vi "Device Label to Configuration.vi"(8 "error in (no error)":errorcluster, 10 "Ring Labels":string[](array[string]), 11 "UI in":T1 {"KH"."Channel" items=["A 1"]}) -> (0 "error out":errorcluster, 3 "UI out":T1 {"KH"."Channel" items=["A 1"]})   [LabVIEW 2016, in "Control Experiment UI.lvclass"]
uses:
  Control Experiment UI.lvclass
  Typedefs/UI Channels--Cluster.ctl
  Typedefs/UI Channels.AI--Cluster.ctl
  Typedefs/UI Channels.Device--Cluster.ctl
  Control Experiment SM/Typedefs/KH Mode-enum.ctl
  Typedefs/UI Channels.KH--Cluster.ctl
  <userlib>/LevyLab/Krohn Hite 7008/typedefs/Input Configuration-Enum.ctl
  <userlib>/LevyLab/Krohn Hite 7008/typedefs/Gain-Enum.ctl
  <userlib>/LevyLab/Krohn Hite 7008/typedefs/Shunt-Enum.ctl
  Typedefs/UI Channels.AO--Cluster.ctl
  <userlib>/LevyLab/Krohn Hite 7008/Instrument.KH7008.lvclass
  Control Experiment SM/Control Experiment SM.lvclass
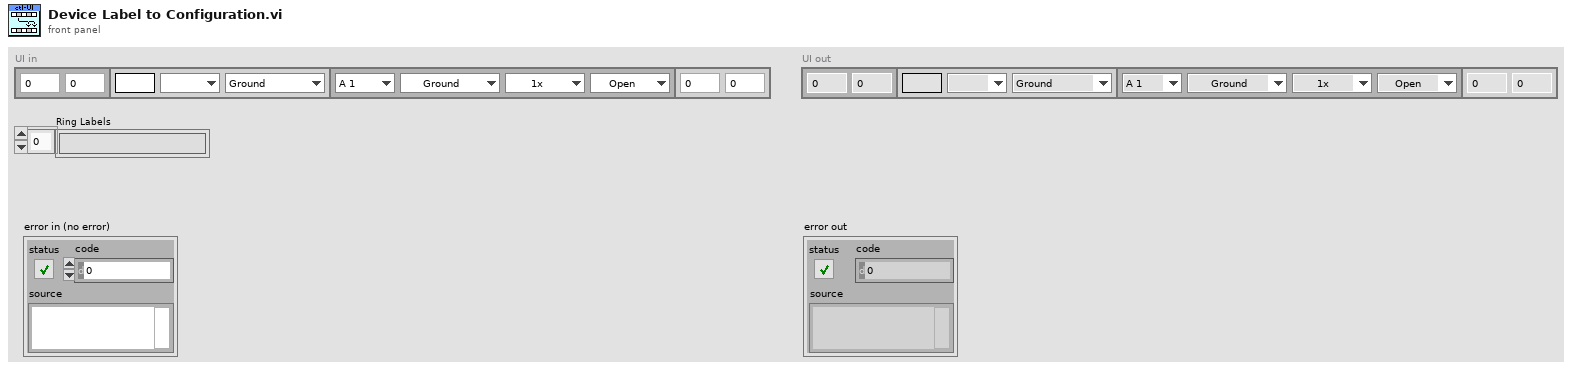
[diagram p1: front panel]
types:
  T1 = typedef "Control Experiment UI.lvclass/UI Channels--Cluster.ctl" = cluster{"AI":T2, "Device":T3, "KH":T5, "AO":T9}
  T2 = typedef "Control Experiment UI.lvclass/UI Channels.AI--Cluster.ctl" = cluster{"Channel":u32, "Gain":dbl}
  T3 = typedef "Control Experiment UI.lvclass/UI Channels.Device--Cluster.ctl" = cluster{"Electrode":string, "Configuration":T4, "Label":u16}
  T4 = typedef "Control Experiment SM.lvclass/KH Mode-enum.ctl" = enum16{"Ground", "Current", "Voltage (SE)", "Voltage (Diff)", "Gate"}
  T5 = typedef "Control Experiment UI.lvclass/UI Channels.KH--Cluster.ctl" = cluster{"Channel":u16, "Configuration":T6, "Gain":T7, "Shunt Resistor":T8}
  T6 = typedef "Instrument.KH7008.lvclass/Input Configuration-Enum.ctl" = enum16{"Ground", "SE+ (-gnd)", "SE- (+gnd)", "Differential"}
  T7 = typedef "Instrument.KH7008.lvclass/Gain-Enum.ctl" = enum16{"1x", "10x", "100x", "1000x"}
  T8 = typedef "Instrument.KH7008.lvclass/Shunt-Enum.ctl" = enum16{"Open", "50 Ohms", "500 Ohms", "5k Ohms", "50k Ohms", "10M Ohm"}
  T9 = typedef "Control Experiment UI.lvclass/UI Channels.AO--Cluster.ctl" = cluster{"Channel":u32, "Gain":dbl}
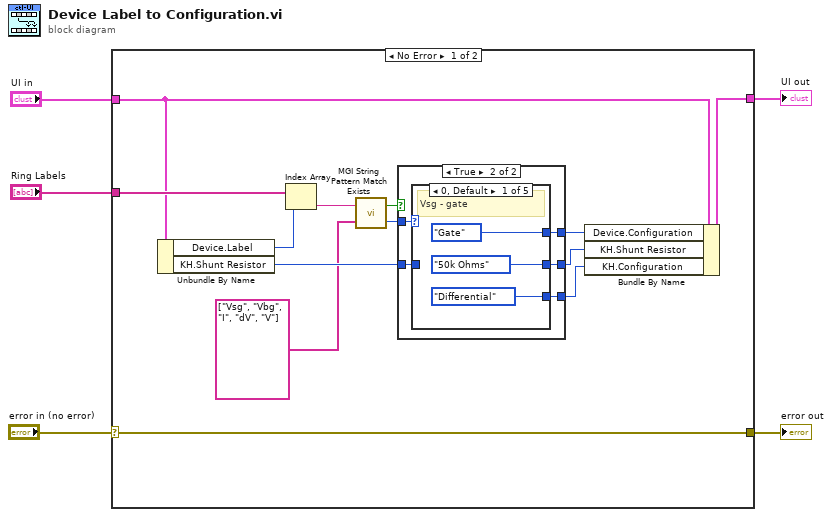
[diagram p0: block diagram]
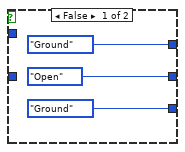
[diagram p2: hidden frame]
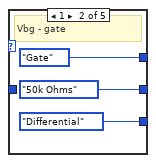
[diagram p3: hidden frame]
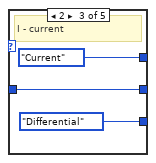
[diagram p4: hidden frame]
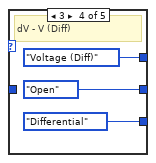
[diagram p5: hidden frame]
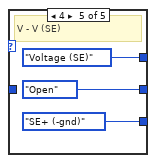
[diagram p6: hidden frame]
diagram:
  n1 = case shown="No Error" "error in (no error)" {
    selector: "error in (no error)" -> [w6 w43]
    tunnel: "Ring Labels" -> [w15 _]
    tunnel: [w14 w42] -> w4
    tunnel: "UI in" -> [w10 w42]
    tunnel: [w6 w43] -> w1
    frame No Error {
      n2 = Unbundle By Name(w10) -> ("Device.Label"=w18:u16, "KH.Shunt Resistor"=w17:T8)
      n3 = Index Array(array=w15, index=w18) -> (element=w8:string)
      n4 = call <userlib>:"MGI String Pattern Match Exists.vi"("Patterns to Try"=string[] ["Vsg", "Vbg", "I", "dV", "V"], "String"=w8) -> ("Index of First Pattern Matched"=w7:i32, "Match Found"=w9:bool)
      n5 = case shown="True" w9 {
        tunnel: w7 -> [_ w26]
        tunnel: [KH_Mode-enum."Ground" ("Enum") w25] -> w11
        tunnel: [Shunt-Enum."Open" ("Shunt Resistor") w24] -> w12
        tunnel: [Input_Configuration-Enum."Ground" ("Input Configuation") w23] -> w13
        tunnel: w17 -> [_ w22]
        frame False {
        }
        frame True {
          n6 = case shown="0, Default" w26 {
            tunnel: [KH_Mode-enum."Gate" ("Enum") KH_Mode-enum."Gate" ("Enum") KH_Mode-enum."Current" ("Enum") KH_Mode-enum."Voltage (Diff)" ("Enum") KH_Mode-enum."Voltage (SE)" ("Enum")] -> w25
            tunnel: [Shunt-Enum."50k Ohms" ("Shunt Resistor") Shunt-Enum."50k Ohms" ("Shunt Resistor") w33 Shunt-Enum."Open" ("Shunt Resistor") Shunt-Enum."Open" ("Shunt Resistor")] -> w24
            tunnel: [Input_Configuration-Enum."Differential" ("Input Configuation") Input_Configuration-Enum."Differential" ("Input Configuation") Input_Configuration-Enum."Differential" ("Input Configuation") Input_Configuration-Enum."Differential" ("Input Configuation") Input_Configuration-Enum."SE+ (-gnd)" ("Input Configuation")] -> w23
            tunnel: w22 -> [_ _ w33 _ _]
            frame 0, Default {
              # "Vsg - gate"
            }
            frame 1 {
              # "Vbg - gate"
            }
            frame 2 {
              # "I - current"
            }
            frame 3 {
              # "dV - V (Diff)"
            }
            frame 4 {
              # "V - V (SE)"
            }
          }
        }
      }
      n7 = Bundle By Name(cluster=w10, "Device.Configuration"=w11, "KH.Shunt Resistor"=w12, "KH.Configuration"=w13) -> (w14:T1)
    }
    frame Error {
    }
  }
  "UI out" <- w4
  "error out" <- w1
